vi "SCL_and_2WML_onlytable2_no_TCP.vi"() -> ()   [LabVIEW 2021]
uses:
  Stub_VIs/WM/wavemeter_server_urls.ctl
  Stub_VIs/WM/IPaddresses.ctl
  <vilib>/Utility/error.llb/DialogType.ctl
panel:
  in  "IP address":T1="cavlab-scancav"
  out "output voltages 2":T2(array[cluster])=[{"saturated"=TRUE, "output voltage"=25.46474000008848}, {"saturated"=TRUE, "output voltage"=1020.26}]
  in  "PID reset SCL":bool[](array[boolean])=[FALSE, FALSE, FALSE, FALSE, FALSE, FALSE]
  out "Wavelength errors 2":dbl[](array[numeric])=[3.909034148819046e-06, 8.932810601436358e-06, 5.7488612128508976e-06, 8.516949606018898e-06]
  in  "Rset/Tset SCL":dbl[](array[numeric])=[38.17, 0.5318, 0.25460629015485653, 0.290618896484375, 0.7917] format="%.4g"
  out "DAC valtage":dbl[](array[numeric])=[-0.5706787109375, 2.4786376953125, 2.645721435546875, 2.03125, 3.220062255859375, 0.0, 0.0, 0.0]
  out "std freq. (MHz)":dbl[](array[numeric])=[0.250954231222493, 0.4256323723137719, 0.20623083149127014, 0.27837611375548527, 0.37702965134812455, 0.3511912133296412, 0.32553785163645144]
  in  "Lock":bool[](array[boolean])=[TRUE, TRUE, TRUE, TRUE, TRUE, FALSE, FALSE]
  out "missing":bool[](array[boolean])
  out "voltage\nsaturated":u32[](array[colorbox])=[1985280, 1985280, 1985280, 1985280, 1985280, 1985280, 1985280, 1985280] caption="saturated"
  in  "stop":bool
  out "actual wavelength 2":dbl[](array[numeric])=[793.918330909034, 866.4525529328106, 850.0353907488612, 854.4437345169496] format="%#.6g"
  in  "locksettings 2":T3(array[cluster])=[{"Wavemeter Channel"=1, "Set Wavelength"=793.9183269999999, "Lock"=FALSE, "Reset"=FALSE, "P Gain"=50.0, "I Gain"=34.0, "D Gain"=0.0}, {"Wavemeter Channel"=2, "Set Wavelength"=866.452544, "Lock"=FALSE, "Reset"=FALSE, "P Gain"=13.0, "I Gain"=70.0, "D Gain"=0.0}, {"Wavemeter Channel"=3, "Set Wavelength"=850.035385, "Lock"=FALSE, "Reset"=FALSE, "P Gain"=45.0, "I Gain"=71.0, "D Gain"=0.0}, {"Wavemeter Channel"=4, "Set Wavelength"=854.443726, "Lock"=FALSE, "Reset"=FALSE, "P Gain"=25.0, "I Gain"=56.0, "D Gain"=0.0}] {"Set Wavelength" format="%.6g"}
  in  "Do not show \nnegative \nwavelengths":bool=TRUE
  in  "Sync":bool
  in  "Clear chart":bool
  in  "Show":bool[](array[boolean])=[TRUE, TRUE, TRUE, TRUE, FALSE, FALSE, FALSE, FALSE]
  out "?":T4(graph)={"[0]"=3.909034148819046e-06, "[1]"=8.932810601436358e-06, "[2]"=5.7488612128508976e-06, "[3]"=8.516949606018898e-06, "[4]"=0.0, "[5]"=0.0, "[6]"=0.0, "[7]"=0.0, "[8]"=0.0}
  in  "P gain SCL":i32[](array[numeric])=[4000, 600, 600, 1000, 400, 300, 1000, 0]
  in  "I gain SCL":i32[](array[numeric])=[1200, 700, 1600, 2100, 1600, 500, 1500, 0]
  in  "Dgain SCL":i32[](array[numeric])=[0, 0, 0, 0, 0, 0, 0, 0]
  in  "Tgain SCL":i32[](array[numeric])=[1, 2, 3, 1, 1, 1, 1, 1]
  in  "peak # SCL":i32[](array[numeric])=[1, 3, 2, 1, 2, 4, 2, 4]
  out "Trigger Time CH1 (us)":T5(graph)={"Time (us)[0]"=38.89, "Time (us)[1]"=249.05, "Time (us)[2]"=138.6, "Time (us)[3]"=0.0, "Time (us)[4]"=0.0, "Time (us)[5]"=0.0, "Time (us)[6]"=0.0, "Time (us)[7]"=0.0, "Time (us)[8]"=0.0}
  out "error":dbl[](array[numeric])=[0.72, 0.000762939453125, -0.00018310546875, 0.0008544921875, -0.001312255859375, 0.209320068359375, 0.791534423828125, 0.0]
  out "Time (us)":dbl[](array[numeric])=[38.89, 249.05, 138.6, 153.03, 351.51, 516.42, 351.34, 433.7]
  out "std time (us)":dbl[](array[numeric])=[0.2647876315010167, 0.39545809138367144, 0.21574020657887225, 0.2053072361717676, 0.1588207820668498, 0.0, 0.20472589938146699, 0.2920737955394419]
  out "R/T":dbl[](array[numeric])=[38.89, 0.532562255859375, 0.25439453125, 0.291473388671875, 0.79034423828125, 0.209320068359375, 0.791534423828125]
  out "T (us)":dbl=395.9
  out "std of T (MHz)":dbl=0.33012019060042547
  out "Error chart":T4(graph)={"[0]"=0.0018186410709775196, "[1]"=0.000762939453125, "[2]"=-0.00018310546875, "[3]"=0.0008544921875, "[4]"=-0.001312255859375, "[5]"=0.209320068359375, "[6]"=0.791534423828125, "[7]"=0.0, "[8]"=0.0}
  out "std chart":T6(graph)={"std freq. (MHz)[0]"=0.250954231222493, "std freq. (MHz)[1]"=0.4256323723137719, "std freq. (MHz)[2]"=0.20623083149127014, "std freq. (MHz)[3]"=0.27837611375548527, "std freq. (MHz)[4]"=0.37702965134812455, "std freq. (MHz)[5]"=0.3511912133296412, "std freq. (MHz)[6]"=0.32553785163645144, "std freq. (MHz)[7]"=0.0, "std freq. (MHz)[8]"=0.0}
  out "Trigger Time CH2 (us)":T5(graph)={"Time (us)[0]"=153.03, "Time (us)[1]"=351.51, "Time (us)[2]"=516.42, "Time (us)[3]"=0.0, "Time (us)[4]"=0.0, "Time (us)[5]"=0.0, "Time (us)[6]"=0.0, "Time (us)[7]"=0.0, "Time (us)[8]"=0.0}
  in  "Lock here SCL":bool[](array[boolean])=[FALSE, FALSE, FALSE, FALSE, FALSE, FALSE, FALSE, FALSE]
  in  "Show 2":bool[](array[boolean])=[TRUE, TRUE, TRUE, TRUE, TRUE, TRUE, FALSE, FALSE]
  out "update ID 3":i32=66220
  in  "Server 2 URL":T7="192.168.0.168"
  out "update ID 2":i32=38594
  out "update ID URL 2":string="dstp://cavlab-lasers/updateid"
  out "Output Voltages URL 2":string="dstp://cavlab-lasers/outputvoltages"
  out "Lock settings URL 2":string="dstp://cavlab-lasers/locksettings"
  out "Current Wavelengths 2":string="dstp://cavlab-lasers/wavelengths_channels"
  out "Dummy Chart":T4(graph)={"[0]"=3.909034148819046e-06, "[1]"=8.932810601436358e-06, "[2]"=5.7488612128508976e-06, "[3]"=8.516949606018898e-06, "[4]"=0.0, "[5]"=0.0, "[6]"=0.0, "[7]"=0.0, "[8]"=0.0}
  # "WML"
  # "nm"
  # "nm"
  # "DAC"
  # "SCL"
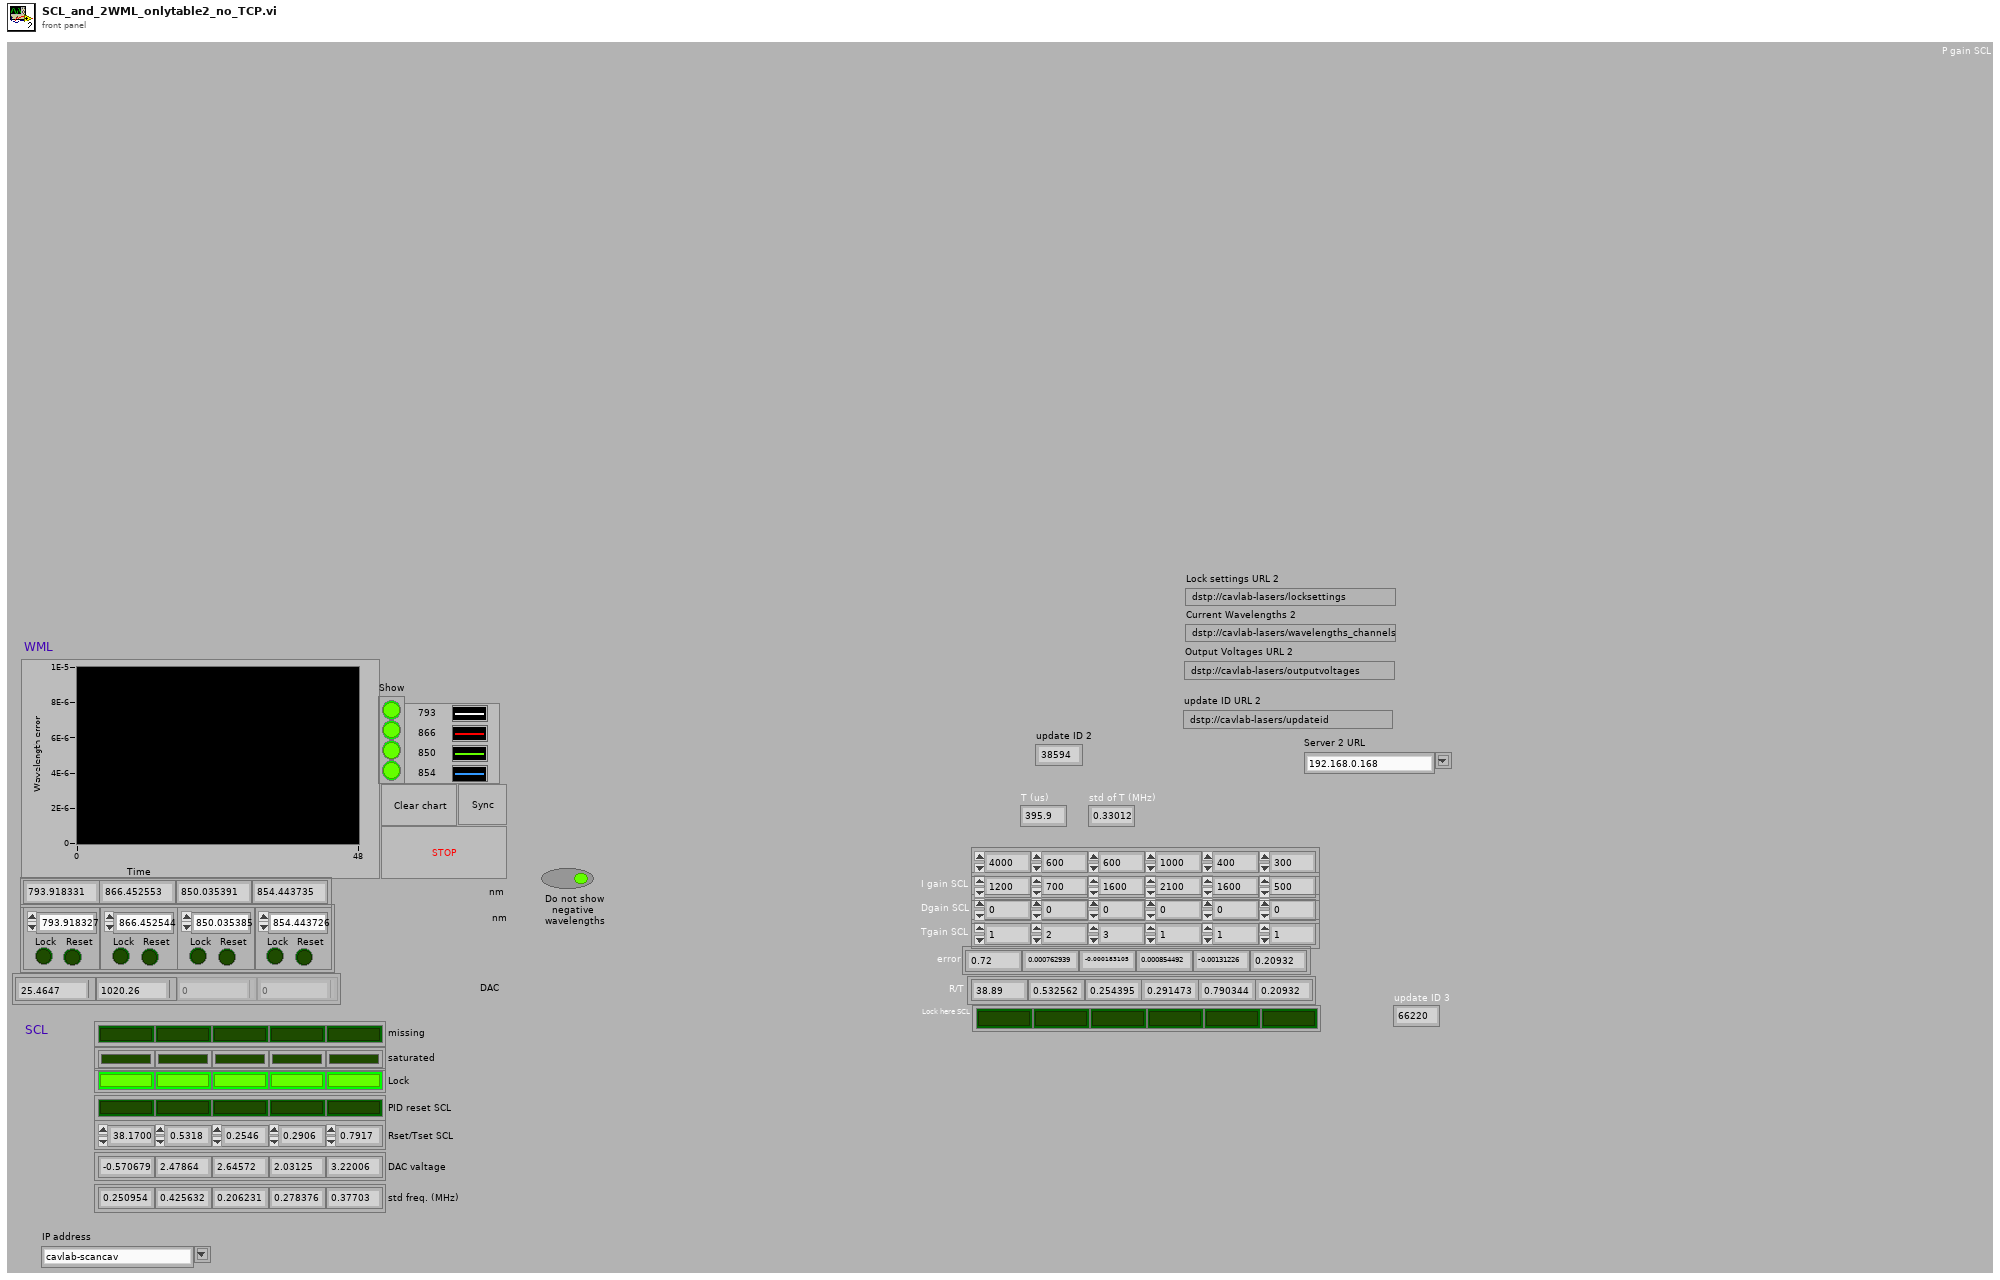
[diagram p1: front panel]
types:
  T1 = typedef "IPaddresses.ctl" = string
  T2 = cluster{"saturated":bool, "output voltage":dbl}[]
  T3 = cluster{"Wavemeter Channel":i32, "Set Wavelength":dbl, "Lock":bool, "Reset":bool, "P Gain":dbl, "I Gain":dbl, "D Gain":dbl}[]
  T4 = cluster{"[0]":dbl, "[1]":dbl, "[2]":dbl, "[3]":dbl, "[4]":dbl, "[5]":dbl, "[6]":dbl, "[7]":dbl, "[8]":dbl}
  T5 = cluster{"Time (us)[0]":dbl, "Time (us)[1]":dbl, "Time (us)[2]":dbl, "Time (us)[3]":dbl, "Time (us)[4]":dbl, "Time (us)[5]":dbl, "Time (us)[6]":dbl, "Time (us)[7]":dbl, "Time (us)[8]":dbl}
  T6 = cluster{"std freq. (MHz)[0]":dbl, "std freq. (MHz)[1]":dbl, "std freq. (MHz)[2]":dbl, "std freq. (MHz)[3]":dbl, "std freq. (MHz)[4]":dbl, "std freq. (MHz)[5]":dbl, "std freq. (MHz)[6]":dbl, "std freq. (MHz)[7]":dbl, "std freq. (MHz)[8]":dbl}
  T7 = typedef "wavemeter_server_urls.ctl" = string
  T8 = cluster{"P gain SCL":i32[], "I gain SCL":i32[], "D gain SCL":i32[], "Tgain SCL":i32[], "Rset/Tset SCL":dbl[], "peak # SCL":i32[], "PID on/off SCL":bool[], "PID reset SCL":bool[], "Lock here SCL":bool[]}
  T9 = enum16{"Read", "Write", "ReadWrite", "BufferedRead", "BufferedReadWrite"}
  T10 = cluster{"Time (us)":dbl[], "R":dbl[], "error":dbl[], "DAC valtage":dbl[], "T (us)":dbl, "std time (us)":dbl[], "std freq. (MHz)":dbl[], "std of T (MHz)":dbl, "missing":bool[], "voltage\nsaturated":u32[]}
  T11 = typedef "DialogType.ctl" = u16
  T12 = cluster{"Wavemeter Channel  ":i32, "Set Wavelength":dbl, "Lock":bool, "Reset":bool, "P Gain":dbl, "I Gain":dbl, "D Gain":dbl}
  T13 = cluster{"Wavemeter Channel  ":i32, "Set Wavelength":dbl, "Lock":bool, "Reset":bool, "P Gain":dbl, "I Gain":dbl, "D Gain":dbl}[]
  T14 = cluster{"Wavelength errors[0]":dbl, "Wavelength errors[1]":dbl, "Wavelength errors[2]":dbl, "Wavelength errors[3]":dbl, "Wavelength errors[4]":dbl, "Wavelength errors[5]":dbl, "Wavelength errors[6]":dbl, "Wavelength errors[7]":dbl, "Wavelength errors[8]":dbl}
  T15 = cluster{"Wavemeter Channel":i32, "Set Wavelength":dbl, "Lock":bool, "Reset":bool, "P Gain":dbl, "I Gain":dbl, "D Gain":dbl}
  T16 = cluster{"[0]":dbl, "[1]":dbl, "[2]":dbl, "[3]":dbl, "[4]":dbl, "[5]":dbl, "[6]":dbl, "[7]":dbl, "[8]":dbl}[]
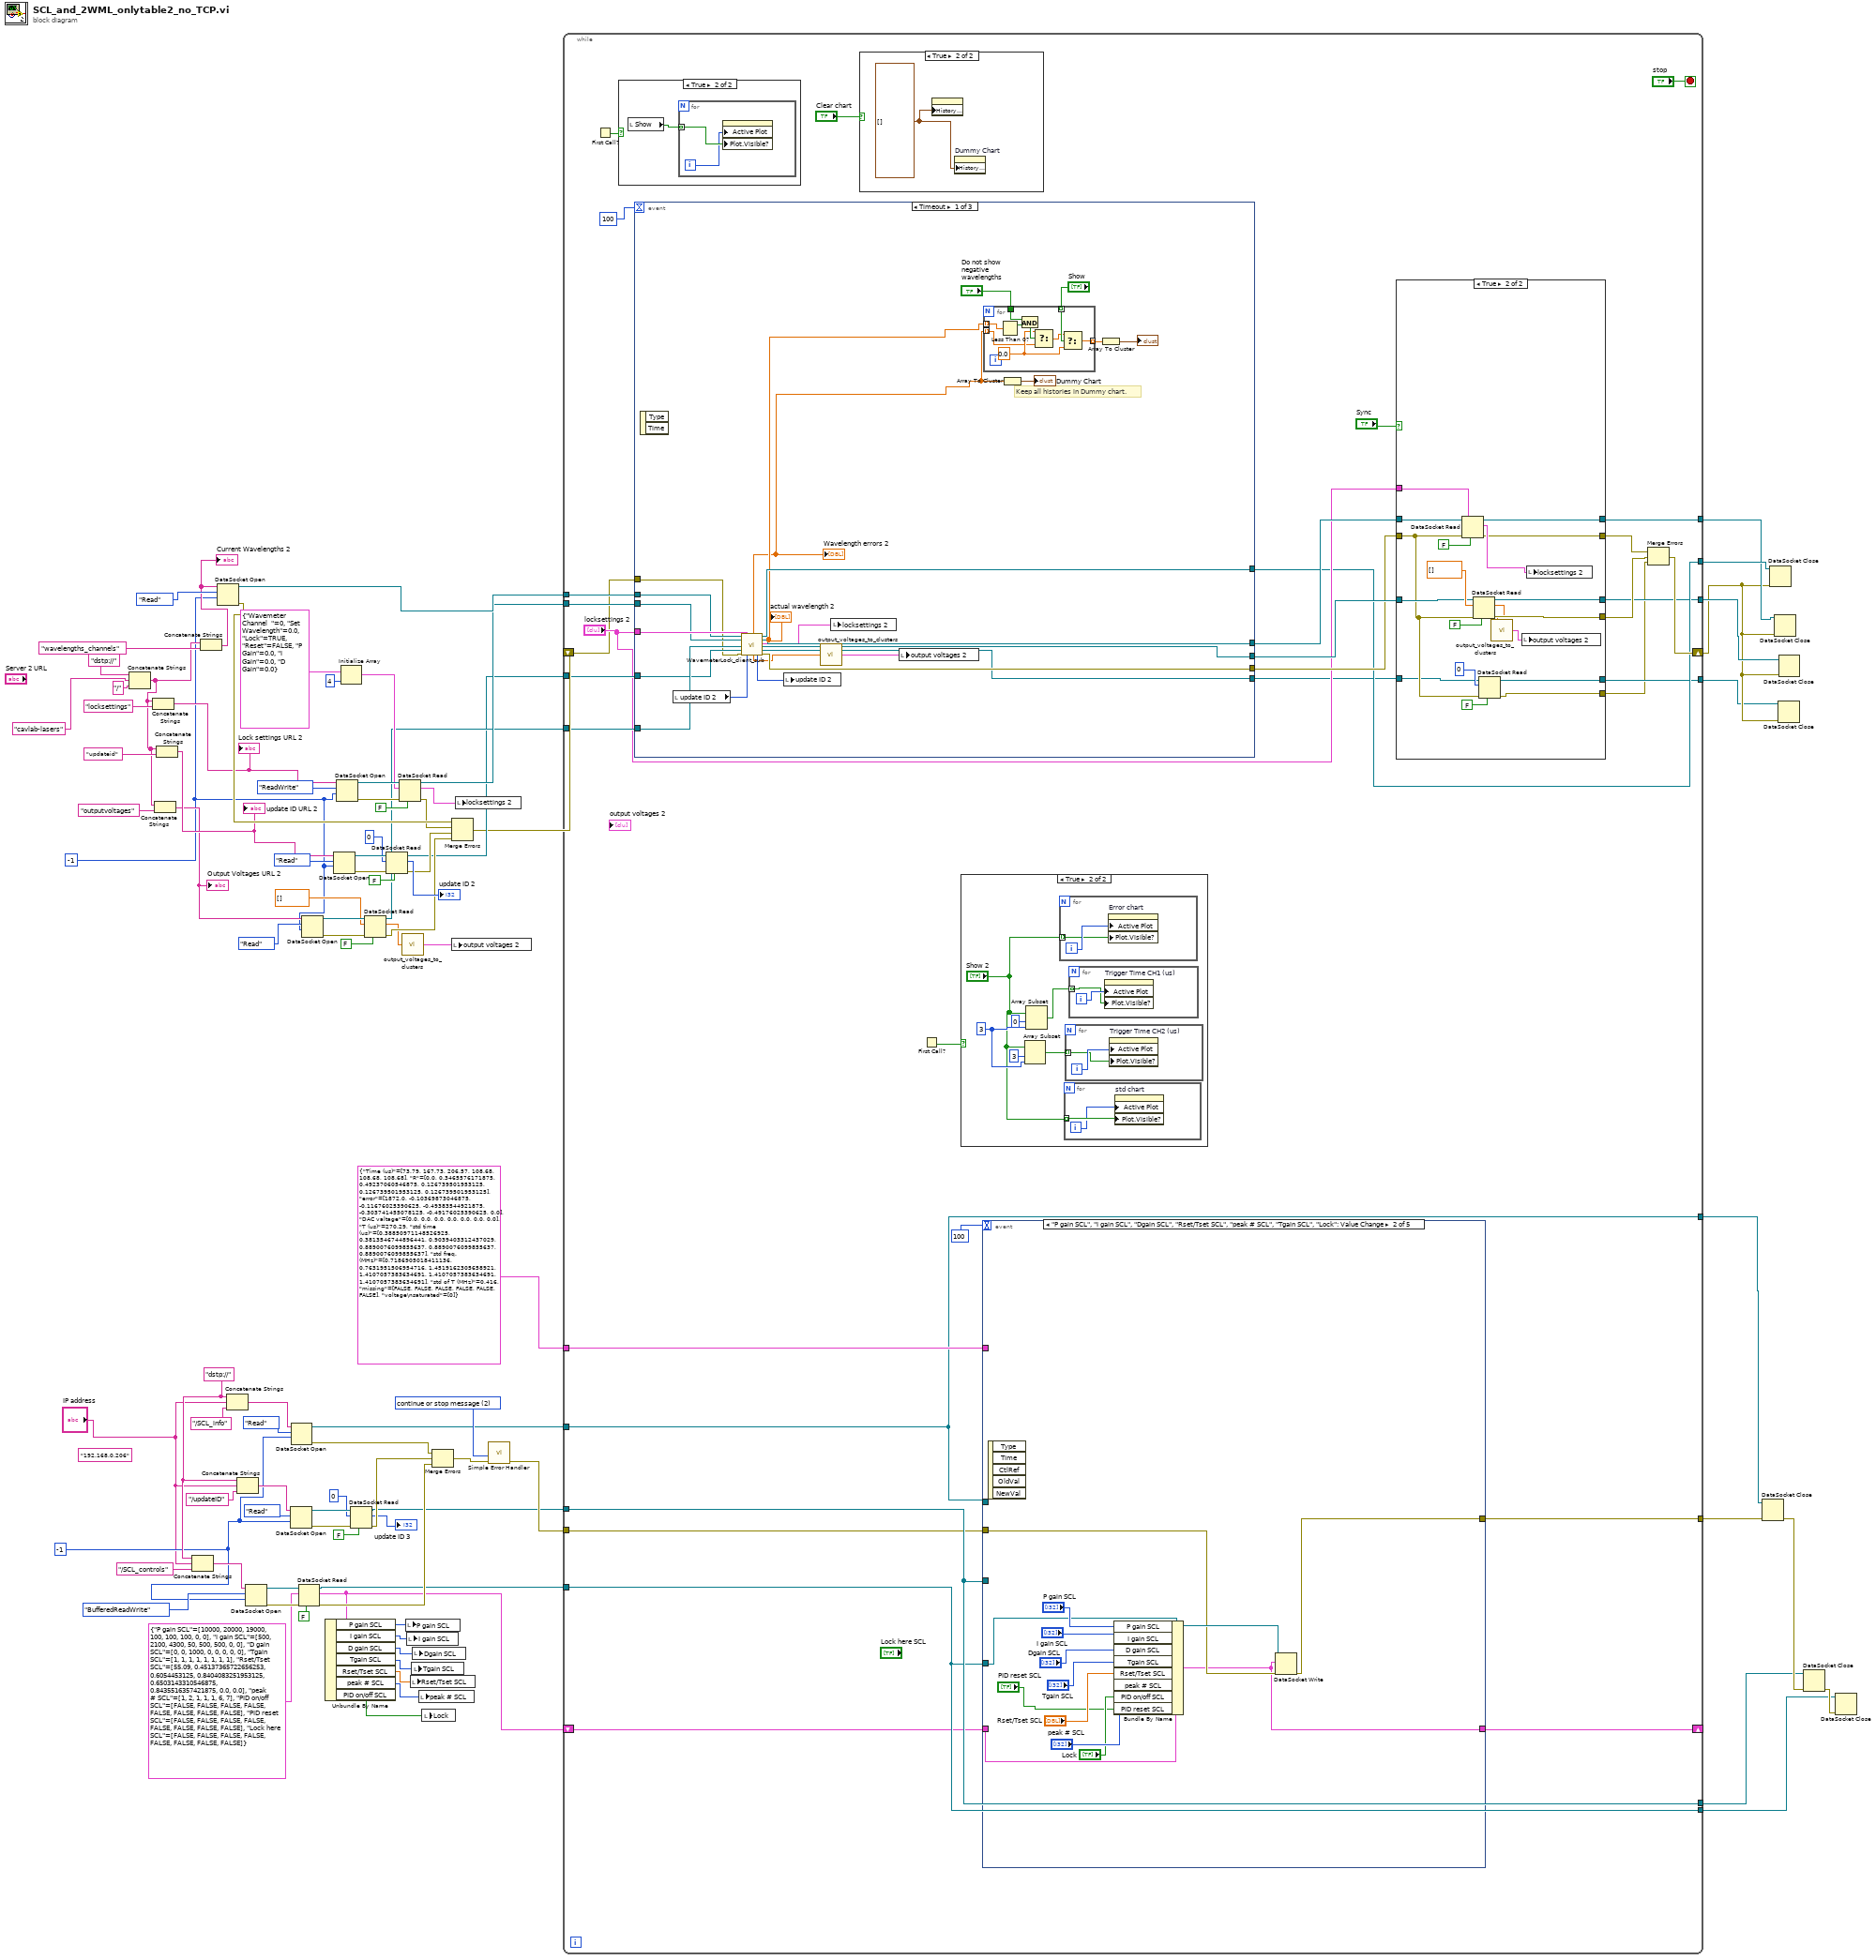
[diagram p0: block diagram]
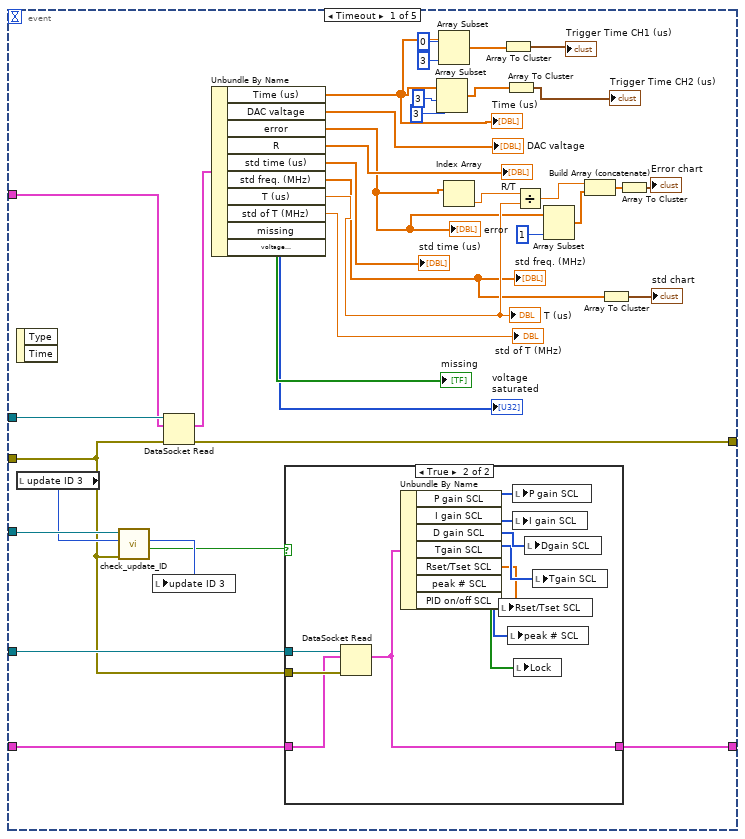
[diagram p2: hidden frame]
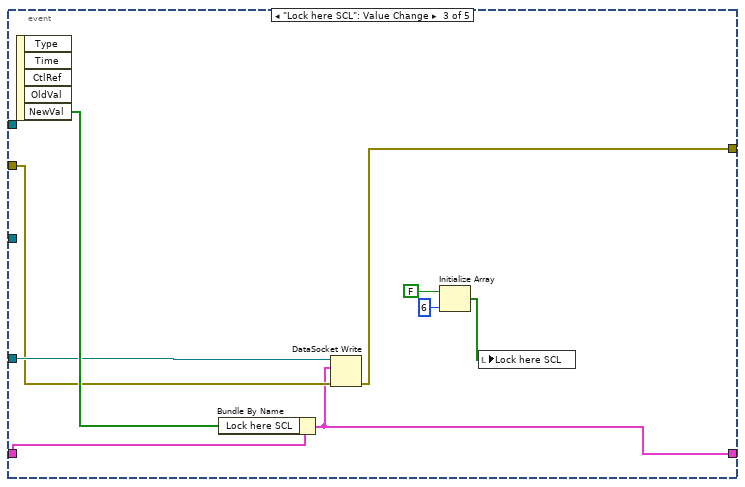
[diagram p4: hidden frame]
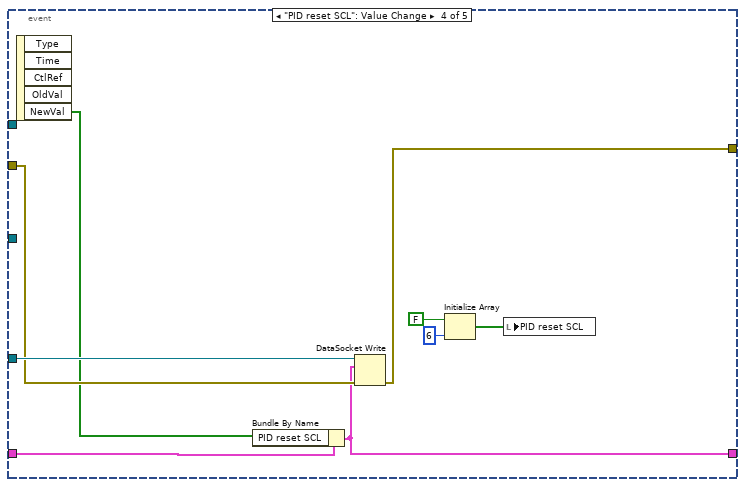
[diagram p5: hidden frame]
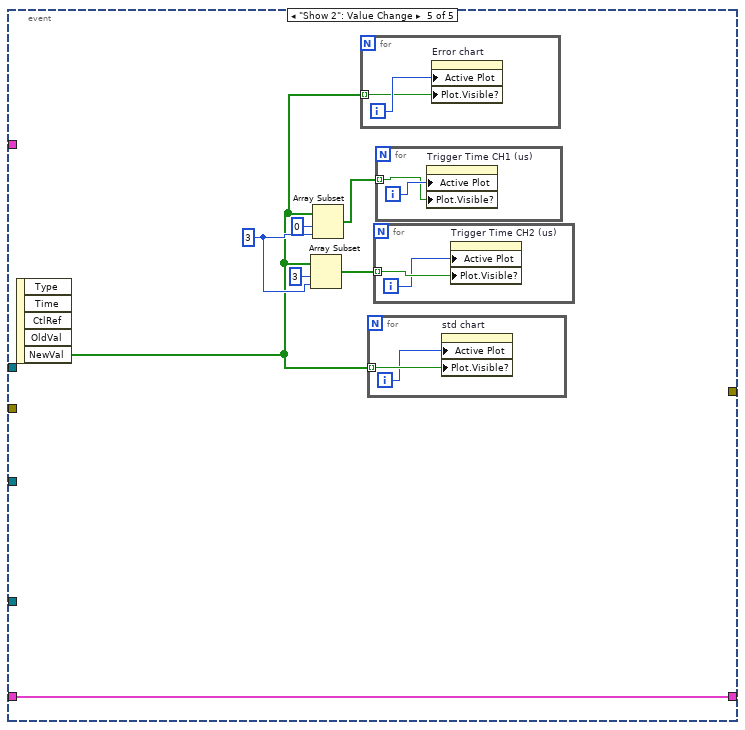
[diagram p6: hidden frame]
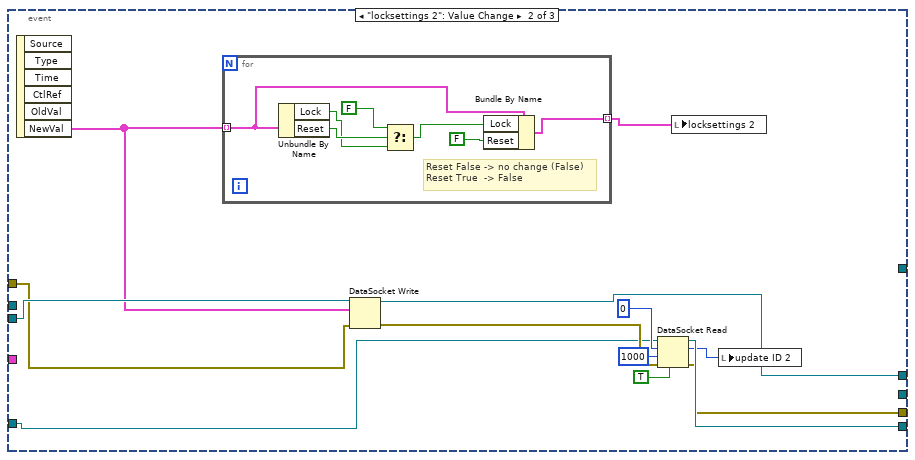
[diagram p11: hidden frame]
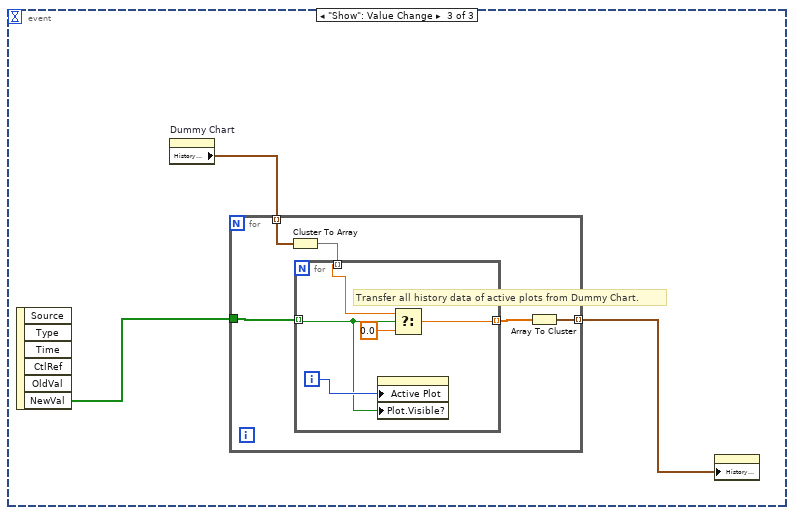
[diagram p12: hidden frame]
diagram:
  w4 = -1
  w5 = -1
  (unwired) "192.168.0.206"
  w44 = T11 2 items=["no dialog", "OK message", "continue or stop message", "OK message + warnings", "continue/stop + warnings"] ("type of dialog (OK msg:1)")
  w35 = "dstp://"
  n1 = Concatenate Strings("dstp://" ("string"), "cavlab-lasers", "/" ("string")) -> (w49:string)
  n2 = Concatenate Strings(w49, "locksettings") -> (w53:string)
  "Lock settings URL 2" <- w53
  n3 = Concatenate Strings(w49, "outputvoltages") -> (w51:string)
  "Output Voltages URL 2" <- w51
  n4 = Concatenate Strings(w49, "updateid" ("string")) -> (w52:string)
  "update ID URL 2" <- w52
  n5 = Concatenate Strings(w35, "IP address", "/SCL_controls") -> (w37:string)
  n6 = Concatenate Strings(w49, "wavelengths_channels" ("string")) -> (w48:string)
  "Current Wavelengths 2" <- w48
  n7 = DataSocket Open(9:w5, 10:T9."Read" ("mode"), 11:w48) -> (0:w74:errorcluster, 3:w70:refnum<k13>)  [unwired: 1 in]
  n8 = Concatenate Strings(w35, "IP address", "/SCL_info") -> (w46:string)
  n9 = Concatenate Strings(w35, "IP address", "/updateID") -> (w42:string)
  n10 = DataSocket Open(9:w4, 10:T9."BufferedReadWrite" ("mode"), 11:w37) -> (0:w28:errorcluster, 3:w29:refnum<k13>)  [unwired: 1 in]
  n11 = DataSocket Open(9:w4, 10:T9."Read" ("mode"), 11:w42) -> (0:w32:errorcluster, 3:w34:refnum<k13>)  [unwired: 1 in]
  n12 = DataSocket Open(9:w4, 10:T9."Read" ("mode"), 11:w46) -> (0:w40:errorcluster, 3:w16:refnum<k13>)  [unwired: 1 in]
  n13 = DataSocket Read(6:FALSE ("wait for updated value (T)"), 8:w28, 10:T8 {"P gain SCL"=[10000, 20000, 19000, 100, 100, 100, 0, 0], "I gain SCL"=[500, 2100, 4300, 50, 500, 500, 0, 0], "D gain SCL"=[0, 0, 1000, 0, 0, 0, 0, 0], "Tgain SCL"=[1, 1, 1, 1, 1, 1, 1, 1], "Rset/Tset SCL"=[55.09, 0.45137365722656253, 0.6054453125, 0.8404083251953125, 0.6503143310546875, 0.8435516357421875, 0.0, 0.0], "peak # SCL"=[1, 2, 1, 1, 1, 6, 7], "PID on/off SCL"=[FALSE, FALSE, FALSE, FALSE, FALSE, FALSE, FALSE, FALSE], "PID reset SCL"=[FALSE, FALSE, FALSE, FALSE, FALSE, FALSE, FALSE, FALSE], "Lock here SCL"=[FALSE, FALSE, FALSE, FALSE, FALSE, FALSE, FALSE, FALSE]}, 11:w29) -> (0:w27:errorcluster, 2:w2:T8, 3:w14:refnum<k13>)  [unwired: 1 in, 4 out]
  n14 = DataSocket Open(9:w5, 10:T9."Read" ("mode"), 11:w51) -> (0:w84:errorcluster, 3:w85:refnum<k13>)  [unwired: 1 in]
  n15 = Unbundle By Name(w2) -> ("P gain SCL"=w23:i32[], "I gain SCL"=w22:i32[], "D gain SCL"=w21:i32[], "Tgain SCL"=w20:i32[], "Rset/Tset SCL"=w1:dbl[], "peak # SCL"=w19:i32[], "PID on/off SCL"=w18:bool[])
  n16 = DataSocket Open(9:w5, 10:T9."Read" ("mode"), 11:w52) -> (0:w78:errorcluster, 3:w79:refnum<k13>)  [unwired: 1 in]
  n17 = DataSocket Open(9:w5, 10:T9."ReadWrite" ("mode"), 11:w53) -> (0:w90:errorcluster, 3:w91:refnum<k13>)  [unwired: 1 in]
  n18 = Initialize Array(T12 {"Wavemeter Channel  "=0, "Set Wavelength"=0.0, "Lock"=TRUE, "Reset"=FALSE, "P Gain"=0.0, "I Gain"=0.0, "D Gain"=0.0}, 4 ("dimension size")) -> (w89:T13)
  n19 = DataSocket Read(6:FALSE ("wait for updated value (T)"), 8:w32, 10:0, 11:w34) -> (0:w31:errorcluster, 2:→"update ID 3":i32, 3:w15:refnum<k13>)  [unwired: 1 in, 4 out]
  n20 = DataSocket Read(6:FALSE ("wait for updated value (T)"), 8:w84, 10:dbl[] [], 11:w85) -> (0:w71:errorcluster, 2:w60:dbl[], 3:w68:refnum<k13>)  [unwired: 1 in, 4 out]
  n21 = DataSocket Read(6:FALSE ("wait for updated value (T)"), 8:w78, 10:0, 11:w79) -> (0:w72:errorcluster, 2:→"update ID 2":i32, 3:w67:refnum<k13>)  [unwired: 1 in, 4 out]
  n22 = DataSocket Read(6:FALSE ("wait for updated value (T)"), 8:w90, 10:w89, 11:w91) -> (0:w73:errorcluster, 2:w87:T13, 3:w69:refnum<k13>)  [unwired: 1 in, 4 out]
  n23 = call "output_voltages_to_clusters.vi"("output voltages"=w60) -> ("output voltage clusters"=w59:T2)
  n24 = local write "P gain SCL"(w23) -> ()
  n25 = local write "I gain SCL"(w22) -> ()
  n26 = local write "Rset/Tset SCL"(w1) -> ()
  n27 = local write "Tgain SCL"(w20) -> ()
  n28 = local write "Dgain SCL"(w21) -> ()
  n29 = local write "peak # SCL"(w19) -> ()
  n30 = local write "Lock"(w18) -> ()
  n31 = Merge Errors(w40, w31, w27) -> (w39:errorcluster)
  n32 = Merge Errors(w74, w73, w72, w71) -> (w66:errorcluster)
  n33 = local write "output voltages 2"(w59) -> ()
  n34 = local write "locksettings 2"(w87) -> ()
  n35 = call <vilib>:"Simple Error Handler.vi"("type of dialog (OK msg:1)"=w44, "error in (no error)"=w39) -> ("error out"=w17:errorcluster)  [unwired: 3 in, 4 out]
  n36 = while {
    tunnel: w70 -> [w122]
    tunnel: w69 -> [w121]
    tunnel: w68 -> [w120]
    tunnel: w67 -> [w119]
    shift-right: [w112] -> w62
    shift-left: w66 -> [w111]
    tunnel: [w110] -> w65
    tunnel: [w109] -> w64
    tunnel: [w108] -> w63
    tunnel: [w106] -> w61
    tunnel: w17 -> [w97]
    tunnel: w16 -> [w95]
    tunnel: w15 -> [w102]
    tunnel: w14 -> [w101]
    tunnel: [w102] -> w11
    tunnel: [w101] -> w10
    shift-right: [w99] -> _
    shift-left: w2 -> [w100]
    tunnel: T10 {"Time (us)"=[73.79, 167.73, 206.57, 108.68, 108.68, 108.68], "R"=[0.0, 0.3465576171875, 0.49237060546875, 0.126739501953125, 0.126739501953125, 0.126739501953125], "error"=[1872.0, -0.10369873046875, -0.11676025390625, -0.49383544921875, -0.303741455078125, -0.49176025390625, 0.0], "DAC valtage"=[0.0, 0.0, 0.0, 0.0, 0.0, 0.0, 0.0], "T (us)"=270.29, "std time (us)"=[0.38850971148526925, 0.3813546744896441, 0.9039403312437029, 0.8890076099855637, 0.8890076099855637, 0.8890076099855637], "std freq. (MHz)"=[0.7186905018411136, 0.7631951506954716, 1.4519162305658921, 1.4107057383634691, 1.4107057383634691, 1.4107057383634691], "std of T (MHz)"=0.416, "missing"=[FALSE, FALSE, FALSE, FALSE, FALSE, FALSE], "voltage\nsaturated"=[0]} -> [w98]
    tunnel: [w96] -> w8
    tunnel: [w95] -> w7
    stop <- "stop" stop-if-true
    n37 = First Call?() -> (First Call?: T/F=w124:bool)
    n38 = case shown="True" w124 {
      frame False {
      }
      frame True {
        n39 = local read "Show"() -> (w260:bool[])
        n40 = for {
          tunnel: w260 -> [w262] mode=indexing
          i -> [w261]
          n41 = property class="WFChart (strict)"("Active Plot"=w261, "Plot.Visible?"=w262) -> ()  [unwired: 2 in, 2 out]
        }
      }
    }
    n42 = event shown="[0] Timeout" {
      selector: _ -> [_ _ _]
      dyn-events: _ -> [_ _ _]
      timeout: 100 -> [_ _ _]
      tunnel: w111 -> [w279 w303 _]
      tunnel: "locksettings 2" -> [w284 _ _]
      tunnel: w122 -> [w283 _ _]
      tunnel: w121 -> [w282 w304 _]
      tunnel: w120 -> [w281 _ _]
      tunnel: w119 -> [w280 w298 _]
      tunnel: [w276 w302 _] -> w118
      tunnel: [w275 _ _] -> w117
      tunnel: [w274 w300 _] -> w116
      tunnel: [w273 _ _] -> w110
      tunnel: [w272 w301 _] -> w107
      event Timeout {
        # "Keep all histories in Dummy chart."
        n43 = event-data() -> ()  [unwired: 1 in, 2 out]
        n44 = local read "update ID 2"() -> (w278:i32)
        n45 = call "WavemeterLock_client_sub.vi"("current wavelengths"=w283, 1:"lock settings"=w282, "output voltages"=w281, 4:"update ID"=w280, "error in (no error)"=w279, 6:"lock settings"=w284, 7:"update ID"=w278) -> ("Wavelength errors"=w264:dbl[], "output voltages"=w270:dbl[], "actual wavelength"=w265:dbl[], "new update ID"=w277:i32, "current wavelength out"=w273:refnum<k13>, "lock settings out"=w276:refnum<k13>, "lock settings new"=w268:T3, "output voltages out"=w275:refnum<k13>, "update ID out"=w272:refnum<k13>, "error out"=w274:errorcluster)  [unwired: 3 in]
        "actual wavelength 2" <- w265
        "Wavelength errors 2" <- w264
        n46 = local write "update ID 2"(w277) -> ()
        n47 = call "output_voltages_to_clusters.vi"("output voltages"=w270) -> ("output voltage clusters"=w269:T2)
        n48 = local write "locksettings 2"(w268) -> ()
        n49 = local write "output voltages 2"(w269) -> ()
        n50 = for {
          tunnel: "Show" -> [w294] mode=indexing
          tunnel: w264 -> [w289] mode=indexing
          tunnel: [w295] -> w271 mode=indexing
          tunnel: "Do not show \nnegative \nwavelengths" -> [w293]
          tunnel: w265 -> [w287] mode=indexing
          w290 = 0.0 ("f")
          n51 = Less Than 0?(x=w287) -> (x < 0?=w292:bool)
          n52 = And(x=w293, y=w292) -> (x .and. y?=w291:bool)
          n53 = Select(t=w290, s=w291, f=w289) -> (s? t:f=w288:dbl)
          n54 = Select(t=w288, s=w294, f=w290) -> (s? t:f=w295:dbl)
        }
        n55 = Array To Cluster(array=w264) -> (cluster=→"Dummy Chart":T14)
        n56 = Array To Cluster(array=w271) -> (cluster=→"?":T4)
      }
      event "locksettings 2": Value Change {
        n57 = event-data() -> ("NewVal"=w296:T3)  [unwired: 1 in, 5 out]
        n58 = for {
          tunnel: w296 -> [w312] mode=indexing
          tunnel: [w309] -> w297 mode=indexing
          # "Reset False -> no change (False)\nReset True  -> False"
          n59 = Unbundle By Name(w312) -> ("Lock"=w313:bool, "Reset"=w315:bool)
          n60 = Select(t=FALSE, s=w315, f=w313) -> (s? t:f=w311:bool)
          n61 = Bundle By Name(cluster=w312, "Lock"=w311, "Reset"=FALSE) -> (w309:T15)
        }
        n62 = DataSocket Write(8:w303, 10:w296, 11:w304) -> (0:w308:errorcluster, 3:w302:refnum<k13>)  [unwired: 1 in, 1 out]
        n63 = DataSocket Read(6:TRUE ("wait for updated value (T)"), 8:w308, 9:1000 ("ms timeout (10000)"), 10:0, 11:w298) -> (0:w300:errorcluster, 2:w299:i32, 3:w301:refnum<k13>)  [unwired: 4 out]
        n64 = local write "locksettings 2"(w297) -> ()
        n65 = local write "update ID 2"(w299) -> ()
      }
      event "Show": Value Change {
        # "Transfer all history data of active plots from Dummy Chart."
        n66 = event-data() -> ("NewVal"=w318:bool[])  [unwired: 1 in, 5 out]
        n67 = property on="Dummy Chart" class="WFChart (strict)"() -> ("History Data"=w317:T16)  [unwired: 2 in, 2 out]
        n68 = for {
          tunnel: w318 -> [w323]
          tunnel: w317 -> [w322] mode=indexing
          tunnel: [w319] -> w316 mode=indexing
          n69 = Cluster To Array(cluster=w322) -> (array=w321:dbl[])
          n70 = for {
            tunnel: w323 -> [w324] mode=indexing
            tunnel: w321 -> [w327] mode=indexing
            tunnel: [w326] -> w320 mode=indexing
            i -> [w325]
            n71 = property class="WFChart (strict)"("Active Plot"=w325, "Plot.Visible?"=w324) -> ()  [unwired: 2 in, 2 out]
            n72 = Select(t=w327, s=w324, f=0.0) -> (s? t:f=w326:dbl)
          }
          n73 = Array To Cluster(array=w320) -> (cluster=w319:T4)
        }
        n74 = property class="WFChart (strict)"("History Data"=w316) -> ()  [unwired: 2 in, 2 out]
      }
    }
    n75 = case shown="True" "Clear chart" {
      frame False {
      }
      frame True {
        w263 = T16 [] ("History Data")
        n76 = property class="WFChart (strict)"("History Data"=w263) -> ()  [unwired: 2 in, 2 out]
        n77 = property on="Dummy Chart" class="WFChart (strict)"("History Data"=w263) -> ()  [unwired: 2 in, 2 out]
      }
    }
    n78 = First Call?() -> (First Call?: T/F=w104:bool)
    n79 = case shown="True" w104 {
      frame False {
      }
      frame True {
        w226 = 3 ("length")
        n80 = Array Subset(array="Show 2", index=3, length=w226) -> (w224:bool[])
        n81 = Array Subset(array="Show 2", index=0, length=w226) -> (w225:bool[])
        n82 = for {
          tunnel: "Show 2" -> [w229] mode=indexing
          i -> [w230]
          n83 = property on="Error chart" class="WFChart (strict)"("Active Plot"=w230, "Plot.Visible?"=w229) -> ()  [unwired: 2 in, 2 out]
        }
        n84 = for {
          tunnel: "Show 2" -> [w232] mode=indexing
          i -> [w231]
          n85 = property on="std chart" class="WFChart (strict)"("Active Plot"=w231, "Plot.Visible?"=w232) -> ()  [unwired: 2 in, 2 out]
        }
        n86 = for {
          tunnel: w224 -> [w233] mode=indexing
          i -> [w234]
          n87 = property on="Trigger Time CH2 (us)" class="WFChart (strict)"("Active Plot"=w234, "Plot.Visible?"=w233) -> ()  [unwired: 2 in, 2 out]
        }
        n88 = for {
          tunnel: w225 -> [w235] mode=indexing
          i -> [w236]
          n89 = property on="Trigger Time CH1 (us)" class="WFChart (strict)"("Active Plot"=w236, "Plot.Visible?"=w235) -> ()  [unwired: 2 in, 2 out]
        }
      }
    }
    n90 = event shown="[1] \"P gain SCL\", \"I gain SCL\", \"Dgain SCL\", \"Rset/Tset SCL\", \"peak # SCL\", \"Tgain SCL\", \"Lock\": Value Change" {
      selector: _ -> [_ _ _ _ _]
      dyn-events: _ -> [_ _ _ _ _]
      timeout: 100 -> [_ _ _ _ _]
      tunnel: w95 -> [w164 _ _ _ _]
      tunnel: w97 -> [w155 w181 w195 w206 _]
      tunnel: w98 -> [w161 _ _ _ _]
      tunnel: [w160 w179 w194 w199 _] -> w96
      tunnel: w102 -> [w159 _ _ _ _]
      tunnel: w101 -> [w156 w182 w196 w207 _]
      tunnel: w100 -> [w154 w189 w198 w205 w208]
      tunnel: [w149 w178 w193 w203 w208] -> w99
      event Timeout {
        n91 = event-data() -> ()  [unwired: 1 in, 2 out]
        n92 = local read "update ID 3"() -> (w158:i32)
        n93 = call "check_update_ID.vi"("error in (no error)"=w155, "previous ID"=w158, "DataSocket Refnum"=w159) -> ("changed?"=w128:bool, "current ID"=w157:i32)  [unwired: 5 in, 2 out]
        n94 = local write "update ID 3"(w157) -> ()
        n95 = DataSocket Read(8:w155, 10:w161, 11:w164) -> (0:w160:errorcluster, 2:w163:T10)  [unwired: 2 in, 5 out]
        n96 = Unbundle By Name(w163) -> ("Time (us)"=w133:dbl[], "DAC valtage"=→"DAC valtage":dbl[], "error"=w144:dbl[], "R"=→"R/T":dbl[], "std time (us)"=→"std time (us)":dbl[], "std freq. (MHz)"=w138:dbl[], "T (us)"=w145:dbl, "std of T (MHz)"=→"std of T (MHz)":dbl, "missing"=→"missing":bool[], "voltage\nsaturated"=→"voltage\nsaturated":u32[])
        "error" <- w144
        "Time (us)" <- w133
        "std freq. (MHz)" <- w138
        "T (us)" <- w145
        n97 = case shown="True" w128 {
          tunnel: w156 -> [_ w176]
          tunnel: w155 -> [_ w175]
          tunnel: w154 -> [w165 w174]
          tunnel: [w165 w166] -> w149
          frame False {
          }
          frame True {
            n98 = DataSocket Read(8:w175, 10:w174, 11:w176) -> (2:w166:T8)  [unwired: 2 in, 6 out]
            n99 = Unbundle By Name(w166) -> ("P gain SCL"=w173:i32[], "I gain SCL"=w172:i32[], "D gain SCL"=w171:i32[], "Tgain SCL"=w170:i32[], "Rset/Tset SCL"=w169:dbl[], "peak # SCL"=w168:i32[], "PID on/off SCL"=w167:bool[])
            n100 = local write "Rset/Tset SCL"(w169) -> ()
            n101 = local write "peak # SCL"(w168) -> ()
            n102 = local write "P gain SCL"(w173) -> ()
            n103 = local write "I gain SCL"(w172) -> ()
            n104 = local write "Lock"(w167) -> ()
            n105 = local write "Dgain SCL"(w171) -> ()
            n106 = local write "Tgain SCL"(w170) -> ()
          }
        }
        n107 = Array Subset(array=w133, index=3, length=3) -> (w130:dbl[])
        n108 = Array Subset(array=w133, index=0, length=3) -> (w134:dbl[])
        n109 = Index Array(array=w144) -> (element=w146:dbl)  [unwired: 1 in]
        n110 = Array To Cluster(array=w134) -> (cluster=→"Trigger Time CH1 (us)":T4)
        n111 = Array To Cluster(array=w130) -> (cluster=→"Trigger Time CH2 (us)":T4)
        n112 = Divide(x=w146, y=w145) -> (x/y=w141:dbl)
        n113 = Array Subset(array=w144, index=1) -> (w142:dbl[])  [unwired: 1 in]
        n114 = Build Array (concatenate)(w141, w142) -> (w140:dbl[])
        n115 = Array To Cluster(array=w138) -> (cluster=→"std chart":T6)
        n116 = Array To Cluster(array=w140) -> (cluster=→"Error chart":T4)
      }
      event "P gain SCL", "I gain SCL", "Dgain SCL", "Rset/Tset SCL", "peak # SCL", "Tgain SCL", "Lock": Value Change {
        n117 = event-data() -> ()  [unwired: 1 in, 5 out]
        n118 = Bundle By Name(cluster=w189, "P gain SCL"="P gain SCL", "I gain SCL"="I gain SCL", "D gain SCL"="Dgain SCL", "Tgain SCL"="Tgain SCL", "Rset/Tset SCL"="Rset/Tset SCL", "peak # SCL"="peak # SCL", "PID on/off SCL"="Lock", "PID reset SCL"="PID reset SCL") -> (w178:T8)
        n119 = DataSocket Write(8:w181, 10:w178, 11:w182) -> (0:w179:errorcluster)  [unwired: 1 in, 2 out]
      }
      event "Lock here SCL": Value Change {
        n120 = event-data() -> ("NewVal"=w197:bool[])  [unwired: 1 in, 4 out]
        n121 = Bundle By Name(cluster=w198, "Lock here SCL"=w197) -> (w193:T8)
        n122 = DataSocket Write(8:w195, 10:w193, 11:w196) -> (0:w194:errorcluster)  [unwired: 1 in, 2 out]
        n123 = Initialize Array(FALSE, 6 ("dimension size")) -> (w190:bool[])
        n124 = local write "Lock here SCL"(w190) -> ()
      }
      event "PID reset SCL": Value Change {
        n125 = event-data() -> ("NewVal"=w204:bool[])  [unwired: 1 in, 4 out]
        n126 = Bundle By Name(cluster=w205, "PID reset SCL"=w204) -> (w203:T8)
        n127 = DataSocket Write(8:w206, 10:w203, 11:w207) -> (0:w199:errorcluster)  [unwired: 1 in, 2 out]
        n128 = Initialize Array(FALSE, 6 ("dimension size")) -> (w200:bool[])
        n129 = local write "PID reset SCL"(w200) -> ()
      }
      event "Show 2": Value Change {
        w212 = 3 ("length")
        n130 = event-data() -> ("NewVal"=w209:bool[])  [unwired: 1 in, 4 out]
        n131 = Array Subset(array=w209, index=3, length=w212) -> (w210:bool[])
        n132 = Array Subset(array=w209, index=0, length=w212) -> (w211:bool[])
        n133 = for {
          tunnel: w209 -> [w215] mode=indexing
          i -> [w216]
          n134 = property on="Error chart" class="WFChart (strict)"("Active Plot"=w216, "Plot.Visible?"=w215) -> ()  [unwired: 2 in, 2 out]
        }
        n135 = for {
          tunnel: w209 -> [w220] mode=indexing
          i -> [w219]
          n136 = property on="std chart" class="WFChart (strict)"("Active Plot"=w219, "Plot.Visible?"=w220) -> ()  [unwired: 2 in, 2 out]
        }
        n137 = for {
          tunnel: w210 -> [w218] mode=indexing
          i -> [w217]
          n138 = property on="Trigger Time CH2 (us)" class="WFChart (strict)"("Active Plot"=w217, "Plot.Visible?"=w218) -> ()  [unwired: 2 in, 2 out]
        }
        n139 = for {
          tunnel: w211 -> [w221] mode=indexing
          i -> [w222]
          n140 = property on="Trigger Time CH1 (us)" class="WFChart (strict)"("Active Plot"=w222, "Plot.Visible?"=w221) -> ()  [unwired: 2 in, 2 out]
        }
      }
    }
    n141 = case shown="True" "Sync" {
      tunnel: w118 -> [w240 w256]
      tunnel: w117 -> [w239 w255]
      tunnel: w116 -> [w238 w246]
      tunnel: "locksettings 2" -> [_ w253]
      tunnel: [w238 w252] -> w114
      tunnel: [w238 w251] -> w113
      tunnel: [w240 w250] -> w109
      tunnel: [w239 w249] -> w108
      tunnel: w107 -> [w237 w245]
      tunnel: [w237 w244] -> w106
      tunnel: [w238 w243] -> w105
      frame False {
      }
      frame True {
        n142 = DataSocket Read(6:FALSE ("wait for updated value (T)"), 8:w246, 10:w253, 11:w256) -> (0:w252:errorcluster, 2:w254:T3, 3:w250:refnum<k13>)  [unwired: 1 in, 4 out]
        n143 = DataSocket Read(6:FALSE ("wait for updated value (T)"), 8:w246, 10:dbl[] [], 11:w255) -> (0:w251:errorcluster, 2:w242:dbl[], 3:w249:refnum<k13>)  [unwired: 1 in, 4 out]
        n144 = DataSocket Read(6:FALSE ("wait for updated value (T)"), 8:w246, 10:0, 11:w245) -> (0:w243:errorcluster, 3:w244:refnum<k13>)  [unwired: 1 in, 5 out]
        n145 = call "output_voltages_to_clusters.vi"("output voltages"=w242) -> ("output voltage clusters"=w241:T2)
        n146 = local write "output voltages 2"(w241) -> ()
        n147 = local write "locksettings 2"(w254) -> ()
      }
    }
    n148 = Merge Errors(w114, w113, w105) -> (w112:errorcluster)
  }
  n149 = DataSocket Close(8:w8, 11:w7) -> (0:w12:errorcluster)  [unwired: 1 in, 1 out]
  n150 = DataSocket Close(8:w62, 11:w65) -> ()  [unwired: 1 in, 2 out]
  n151 = DataSocket Close(8:w62, 11:w64) -> ()  [unwired: 1 in, 2 out]
  n152 = DataSocket Close(8:w62, 11:w61) -> ()  [unwired: 1 in, 2 out]
  n153 = DataSocket Close(8:w62, 11:w63) -> ()  [unwired: 1 in, 2 out]
  n154 = DataSocket Close(8:w12, 11:w11) -> (0:w13:errorcluster)  [unwired: 1 in, 1 out]
  n155 = DataSocket Close(8:w13, 11:w10) -> ()  [unwired: 1 in, 2 out]
